vi "SQL_query.vi"(3 "error in (no error)":errorcluster, 4 "SQL query":string, 5 "联机模式":enum16{"单机", "追溯"}(ring)=enum."追溯") -> (0 "error out":errorcluster, 1 "data":string[][](array[string]))   [LabVIEW 2020]
uses:
  <vilib>/addons/database/Connection.llb/DB Tools Open Connec (String).vi
  <vilib>/addons/database/Connection.llb/Conn Execute.vi
  <vilib>/addons/database/Recordset.llb/Rec Fetch Recordset Data (R).vi
  <vilib>/addons/database/Recordset.llb/Rec Destroy - Connection.vi
  <vilib>/addons/database/NI_Database_API.lvlib
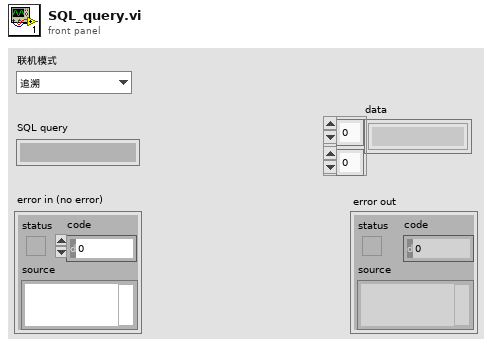
[diagram p1: front panel]
types:
  T1 = typedef "NI_Database_API.lvlib/Conn ObjectReference.ctl" = refnum<k1>
  T2 = typedef "NI_Database_API.lvlib/Rec ObjectReference.ctl" = refnum<k1>
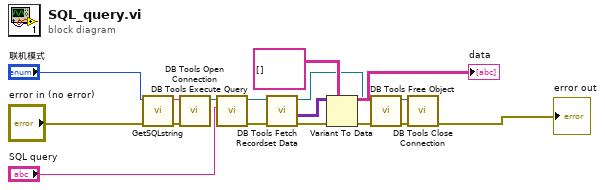
[diagram p0: block diagram]
diagram:
  n1 = call "GetSQLstring.vi"("错误输入"="error in (no error)", "联机模式"="联机模式") -> ("错误输出"=w7:errorcluster, "连接字符串"=w9:string)  [unwired: 8 in]
  n2 = call-poly <vilib>:"DB Tools Open Connection.vi"("error in (no error)"=w7, "connection information"=w9) -> ("connection reference"=w11:T1)  [unwired: 6 in, 1 out]
  n3 = call-poly <vilib>:"DB Tools Execute Query.vi"("SQL query"="SQL query", "connection reference"=w11) -> ("error out"=w17:errorcluster, "recordset reference"=w16:T2)  [unwired: 6 in]
  n4 = call-poly <vilib>:"DB Tools Fetch Recordset Data.vi"("error in (no error)"=w17, "recordset reference"=w16) -> ("error out"=w15:errorcluster, "recordset data"=w14:variant[][], "recordset reference out"=w5:T2)  [unwired: 3 in]
  n5 = Variant To Data(error in=w15, type=string[][] [], Variant=w14) -> (data=→"data":string[][], error out=w4:errorcluster)
  n6 = call-poly <vilib>:"DB Tools Free Object.vi"("error in (no error)"=w4, "recordset reference"=w5) -> ("error out"=w2:errorcluster, "connection reference"=w3:T1)  [unwired: 8 in]
  n7 = call <vilib>:"DB Tools Close Connection.vi"("error in (no error)"=w2, "connection reference"=w3) -> ("error out"=→"error out":errorcluster)  [unwired: 5 in]
